vi "Log_1.vi"(7 "log level":T1=enum."Critical", 8 "error in":errorcluster, 9 "data (null)":variant, 10 "message":string, 11 "logger in":refnum<class "Logger.lvclass">) -> (0 "error out":errorcluster, 3 "logger out":refnum<class "Logger.lvclass">)   [LabVIEW 2018]
uses:
  src/api/Log Levels.ctl
  src/api/logger_class/Logger.lvclass
  src/api/GLog.lvlib
panel:
  # "Connector Pane"
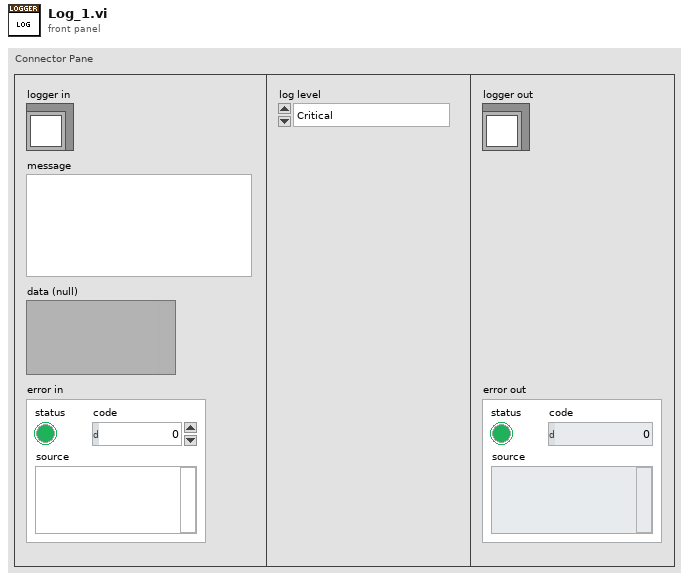
[diagram p1: front panel]
types:
  T1 = typedef "GLog.lvlib/Log Levels.ctl" = enum16{"Trace", "Debug", "Info", "Warning", "Error", "Critical"}
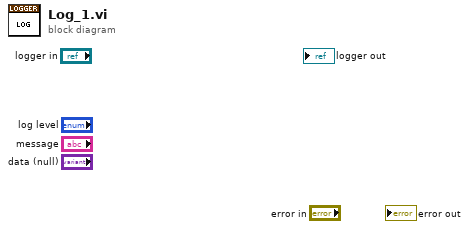
[diagram p0: block diagram]
diagram:
